vi "Test Buffer to ARGB.vi"(8 "error in (no error)":errorcluster, 11 "Test Case In":refnum<class "01_Image.lvclass">) -> (0 "error out":errorcluster, 3 "Test Case Out":refnum<class "01_Image.lvclass">)   [LabVIEW 2020, in "test.lvlib" / "01_Image.lvclass"]
uses:
  01_Image.lvclass
  C:/Program Files (x86)/National Instruments/LabVIEW 2026/vi.lib/Astemes/LUnit/Test Case.lvclass
  image/Buffer Information.ctl
  image/Raw Memory Information Dimension.ctl
  common/Image Size (Integer).ctl
  <vilib>/Astemes/LUnit/Test Case.lvclass/Test Case.ctl
  image/New Image (Greyscale Preallocated).vi
  image/Copy Buffer to Image (Custom Stride Greyscale).vi
  4993e8ee-a06a-463a-9684-69129f64d5ce.vi
  image/New Image (ARGB Preallocated).vi
  image/Copy Buffer to Image (Custom Stride ARGB).vi
  4d87dc2e-cd37-40f4-999a-c108778696d8.vi
  image/Copy Array to Image.vi
  image/Copy Array to Image (Greyscale).vi
  image/New Image (Greyscale Preallocated).vi/6598b9e0-8a08-46f5-91fd-ca1b87217137.vi
  image/Copy Buffer to Image (Custom Stride Greyscale).vi/f11fe23a-4bac-4ce6-b593-80dfc143e0fd.vi
  <vilib>/Astemes/LUnit/Core/LUnit Test Case/Private/Append Pass Result.vi
  <vilib>/Astemes/LUnit/Core/LUnit Test Case/Private/Append Fail Result.vi
  4993e8ee-a06a-463a-9684-69129f64d5ce.vi/9c5d11cd-9439-4240-a1ee-d9baace9c924.vi
  image/Copy Array to Image (ARGB).vi
  image/New Image (ARGB Preallocated).vi/3321fa97-f432-4e1e-8db9-a0df79aed21b.vi
  image/ARGB Colour to U32 Pixel Value.vi
  image/Copy Buffer to Image (Custom Stride ARGB).vi/f11fe23a-4bac-4ce6-b593-80dfc143e0fd.vi
  4d87dc2e-cd37-40f4-999a-c108778696d8.vi/9c5d11cd-9439-4240-a1ee-d9baace9c924.vi
  <vilib>/Astemes/LUnit/Core/LUnit Test Case/Private/Run In UI.vi
  <vilib>/Utility/error.llb/Clear Errors.vi
  <vilib>/Utility/error.llb/Error Cluster From Error Code.vi
  <vilib>/picture/pixmap.llb/Flatten Pixmap.vi
  image/image.lvlib
  common/common.lvlib
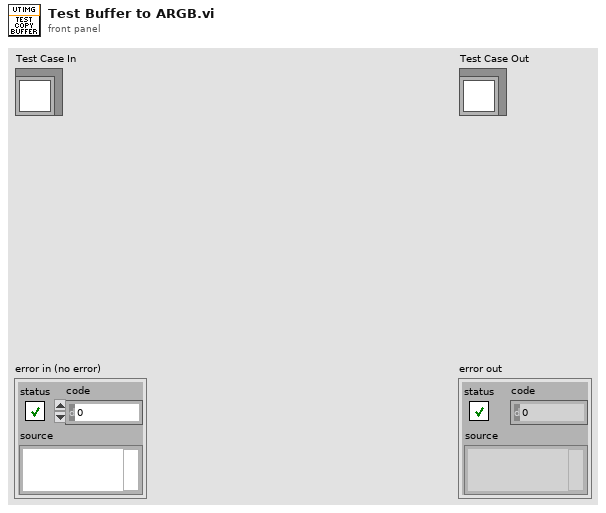
[diagram p1: front panel]
types:
  T1 = enum16{"big-endian, network order", "native, host order", "little-endian"}
  T2 = typedef "image.lvlib/Buffer Information.ctl" = cluster{"Dimension 0":T3, "Dimension 1":T3}
  T3 = typedef "image.lvlib/Raw Memory Information Dimension.ctl" = cluster{"Size":u16, "Stride":i32}
  T4 = typedef "common.lvlib/Image Size (Integer).ctl" = cluster{"Width":u16, "Height":u16}
  T5 = typedef "image.lvlib/Greyscale Image.ctl" = refnum<data-value>
  T6 = typedef "image.lvlib/ARGB Image.ctl" = refnum<data-value>
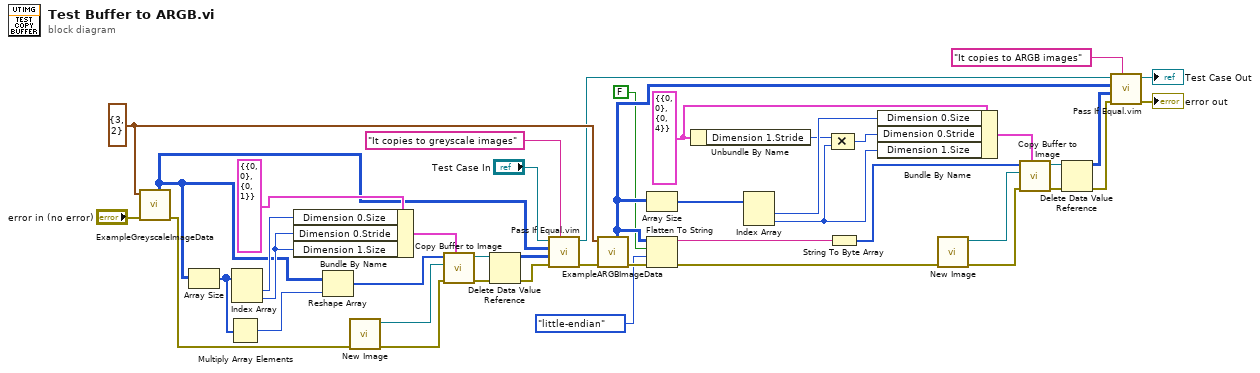
[diagram p0: block diagram]
diagram:
  w11 = T2 {"Dimension 0"={"Size"=0, "Stride"=0}, "Dimension 1"={"Size"=0, "Stride"=4}} ("Buffer Layout")
  w25 = T4 {"Width"=3, "Height"=2} ("Image Size")
  n1 = call "ExampleGreyscaleImageData.vi"("error in (no error)"="error in (no error)", "Image Size"=w25) -> ("error out"=w39:errorcluster, "Greyscale Data"=w28:u8[][])  [unwired: 6 in, 2 out]
  n2 = Array Size(array=w28) -> (size(s)=w37:i32[])
  n3 = Multiply Array Elements(1:w37) -> (0:w42:i32)
  n4 = Index Array(array=w37) -> (element #1=w30:i32, element #2=w29:i32)  [unwired: 2 in]
  n5 = Bundle By Name(cluster=T2 {"Dimension 0"={"Size"=0, "Stride"=0}, "Dimension 1"={"Size"=0, "Stride"=1}} ("Buffer Layout"), "Dimension 0.Size"=w30, "Dimension 0.Stride"=w29, "Dimension 1.Size"=w29) -> (w35:T2)
  n6 = Reshape Array(w28, w42) -> (w41:u8[])
  n7 = call-poly "New Image.vi"("error in (no error)"=w39) -> ("error out"=w38:errorcluster, "Greyscale Image"=w40:T5)  [unwired: 9 in]
  n8 = call-poly "Copy Buffer to Image.vi"("Buffer Layout"=w35, "error in (no error)"=w38, "Greyscale Image Destination in"=w40, "Buffer"=w41) -> ("error out"=w33:errorcluster, "Greyscale Image Destination"=w34:T5)  [unwired: 6 in]
  n9 = Delete Data Value Reference(data value reference=w34, error in=w33) -> (data value=w31:u8[][], error out=w32:errorcluster)
  n10 = call "Pass If Equal.vim"("Description"="It copies to greyscale images", "error in (no error)"=w32, "Actual"=w31, "Expected"=w28, "LUnit Test Case In"="Test Case In") -> ("error out"=w26:errorcluster, "LUnit Test Case Out"=w24:refnum<class "01_Image.lvclass">)  [unwired: 5 in]
  n11 = call "ExampleARGBImageData.vi"("error in (no error)"=w26, "Image Size"=w25) -> ("error out"=w5:errorcluster, "ARGB Array Data"=w6:u32[][])  [unwired: 6 in, 2 out]
  n12 = Array Size(array=w6) -> (size(s)=w13:i32[])
  n13 = Flatten To String(anything=w6, prepend array or string size? (T)=FALSE, byte order (0:big-endian, network order)=T1."little-endian", error in (no error)=w5) -> (data string=w3:string, error out=w4:errorcluster)  [unwired: 1 out]
  n14 = Unbundle By Name(w11) -> ("Dimension 1.Stride"=w9:i32)
  n15 = Index Array(array=w13) -> (element #1=w10:i32, element #2=w7:i32)  [unwired: 2 in]
  n16 = String To Byte Array(string=w3) -> (unsigned byte array=w12:u8[])
  n17 = Compound Arithmetic op=MULTIPLY(w9, w7) -> (w8:i32)
  n18 = Bundle By Name(cluster=w11, "Dimension 0.Size"=w10, "Dimension 0.Stride"=w8, "Dimension 1.Size"=w7) -> (w19:T2)
  n19 = call-poly "New Image.vi"("error in (no error)"=w4) -> ("error out"=w18:errorcluster, "ARGB Image"=w17:T6)  [unwired: 9 in]
  n20 = call-poly "Copy Buffer to Image.vi"("Buffer Layout"=w19, "error in (no error)"=w18, "ARGB Image Destination in"=w17, "Buffer"=w12) -> ("error out"=w21:errorcluster, "ARGB Image Destination"=w20:T6)  [unwired: 6 in]
  n21 = Delete Data Value Reference(data value reference=w20, error in=w21) -> (data value=w14:u32[][], error out=w16:errorcluster)
  n22 = call "Pass If Equal.vim"("Description"="It copies to ARGB images", "error in (no error)"=w16, "Actual"=w14, "Expected"=w6, "LUnit Test Case In"=w24) -> ("error out"=→"error out":errorcluster, "LUnit Test Case Out"=→"Test Case Out":refnum<class "01_Image.lvclass">)  [unwired: 5 in]
